vi "ClearWorkingDirectory.vi"(6 "Status":refnum<vi>, 8 "error in":errorcluster, 11 "Working Path":path) -> (0 "error out":errorcluster, 3 "Working Path Out":path)   [LabVIEW 2022 SP3]
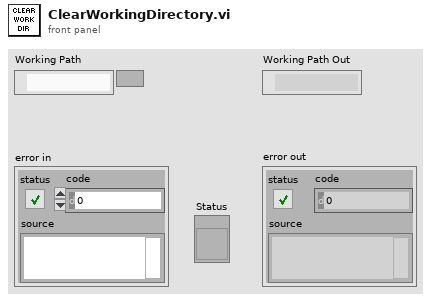
[diagram p1: front panel]
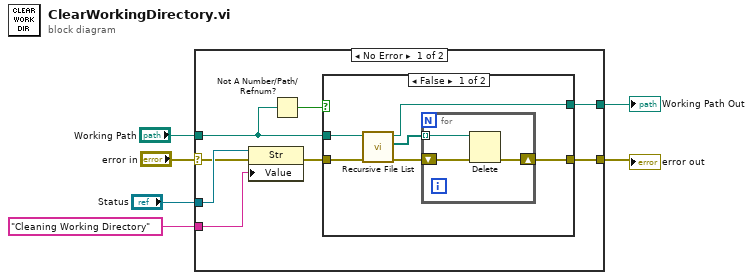
[diagram p0: block diagram]
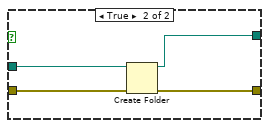
[diagram p2: hidden frame]
diagram:
  n1 = case shown="No Error" "error in" {
    selector: "error in" -> [w7 w29]
    tunnel: "Working Path" -> [w14 w28]
    tunnel: [w13 w28] -> w5
    tunnel: [w11 w29] -> w4
    tunnel: "Status" -> [w9 _]
    tunnel: "Cleaning Working Directory" -> [w8 _]
    frame No Error {
      n2 = property class="Str"(reference=w9, error in=w7, "Value"=w8) -> (error out=w10:errorcluster)  [unwired: 1 out]
      n3 = Not A Number/Path/Refnum?(number/path/refnum=w14) -> (NaN/Path/Refnum?=w12:bool)
      n4 = case shown="False" w12 {
        tunnel: w10 -> [w20 w27]
        tunnel: w14 -> [w17 w26]
        tunnel: [w16 w24] -> w13
        tunnel: [w15 w25] -> w11
        frame False {
          n5 = call <vilib>:"Recursive File List.vi"("error in (no error)"=w20, "Folder Path"=w17) -> ("error out"=w18:errorcluster, "All Files in Dir"=w19:path[], "dup Folder Path"=w16:path)  [unwired: 5 in, 2 out]
          n6 = for {
            tunnel: w19 -> [w23] mode=indexing
            shift-right: [w21] -> w15
            shift-left: w18 -> [w22]
            n7 = Delete(path (use dialog)=w23, error in=w22) -> (error out=w21:errorcluster)  [unwired: 3 in, 2 out]
          }
        }
        frame True {
          n8 = Create Folder(path (use dialog)=w26, error in=w27) -> (created path=w24:path, error out=w25:errorcluster)  [unwired: 1 in, 1 out]
        }
      }
    }
    frame Error {
    }
  }
  "Working Path Out" <- w5
  "error out" <- w4
